vi "Write Program ID.vi"(8 "error in (no error)":errorcluster, 10 "Program ID":string, 11 "User in":refnum<class "User.lvclass">) -> (0 "error out":errorcluster, 3 "User out":refnum<class "User.lvclass">)   [LabVIEW 2018, in "User.lvclass"]
doc: "Este VI escreve na classe o ID do programa."
uses:
  User.lvclass
  User.lvclass/User.ctl
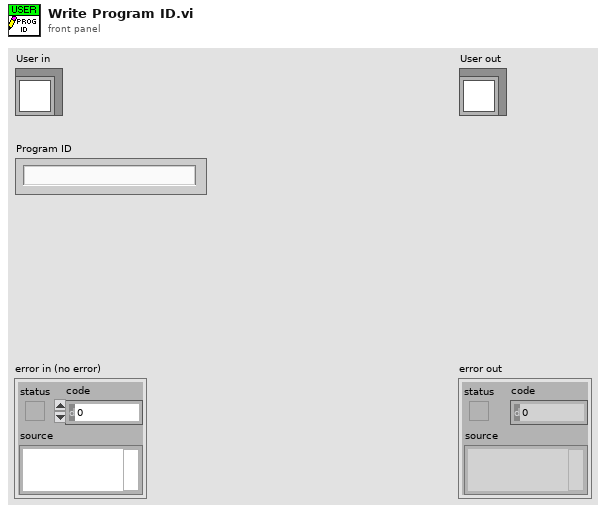
[diagram p1: front panel]
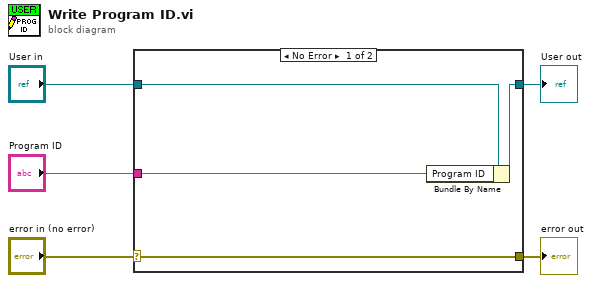
[diagram p0: block diagram]
diagram:
  n1 = case shown="No Error" "error in (no error)" {
    selector: "error in (no error)" -> [w9 w10]
    tunnel: [w9 w10] -> w4
    tunnel: [w7 w11] -> w2
    tunnel: "User in" -> [w8 w11]
    tunnel: "Program ID" -> [w6 _]
    frame No Error {
      n2 = Bundle By Name(cluster=w8, "Program ID"=w6) -> (w7:refnum<class "User.lvclass">)
    }
    frame Error {
    }
  }
  "error out" <- w4
  "User out" <- w2
